vi "Format string to scroll message with time stamp.vi"(8 "error in (no error)":errorcluster, 11 "Status message":string) -> (0 "error out":errorcluster, 2 "Status message out":string, 3 "Status messages accumulated":string)   [LabVIEW 2020]
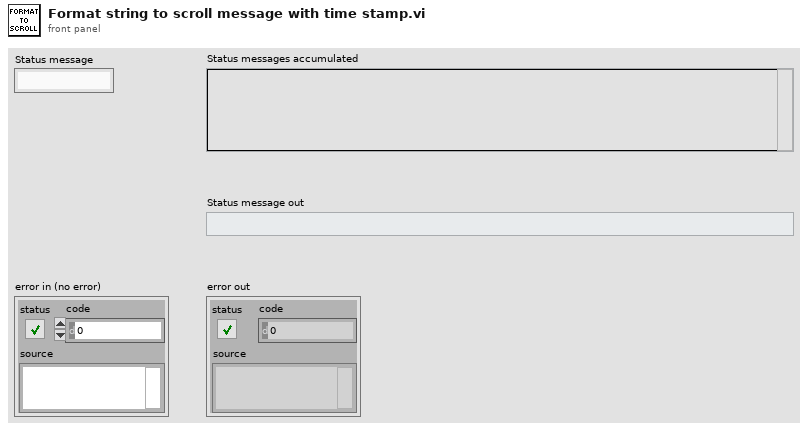
[diagram p1: front panel]
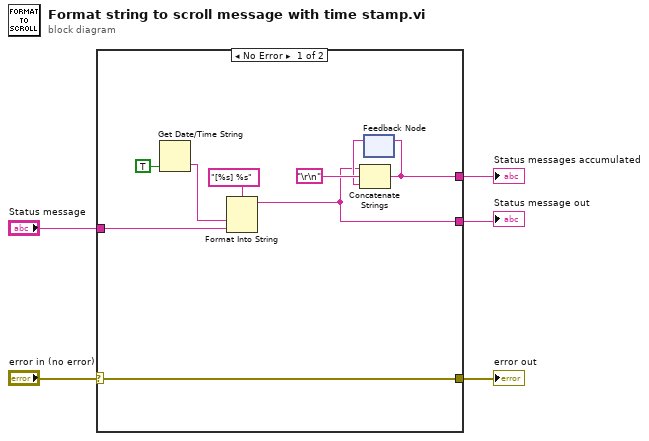
[diagram p0: block diagram]
diagram:
  n1 = case shown="No Error" "error in (no error)" {
    selector: "error in (no error)" -> [w6 w15]
    tunnel: "Status message" -> [w11 w16]
    tunnel: [w9 w16] -> w4
    tunnel: [w7 w16] -> w3
    tunnel: [w6 w15] -> w1
    frame No Error {
      n2 = Get Date/Time String(want seconds? (F)=TRUE) -> (time string=w13:string)  [unwired: 2 in, 1 out]
      n3 = Format Into String(format string="[%s] %s", w13, w11) -> (resulting string=w7:string)  [unwired: 2 in, 1 out]
      n4 = feedback #1() -> (w8:string)  [unwired: 1 in]
      n5 = Concatenate Strings(w7, "\r\n", w8) -> (w9:string)
      n6 = feedback-in #1(w9) -> ()
    }
    frame Error {
    }
  }
  "Status messages accumulated" <- w4
  "error out" <- w1
  "Status message out" <- w3
